vi "GrapFramesRollingBuffer.vi"(0 "object in":refnum<class "Hamamatsu.lvclass">, 5 "error in (no error)":errorcluster) -> (14 "object out":refnum<class "Hamamatsu.lvclass">, 19 "error out":errorcluster)   [LabVIEW 2019, in "Hamamatsu.lvclass"]
uses:
  Hamamatsu.lvclass
  Hamamatsu.lvclass/Hamamatsu.ctl
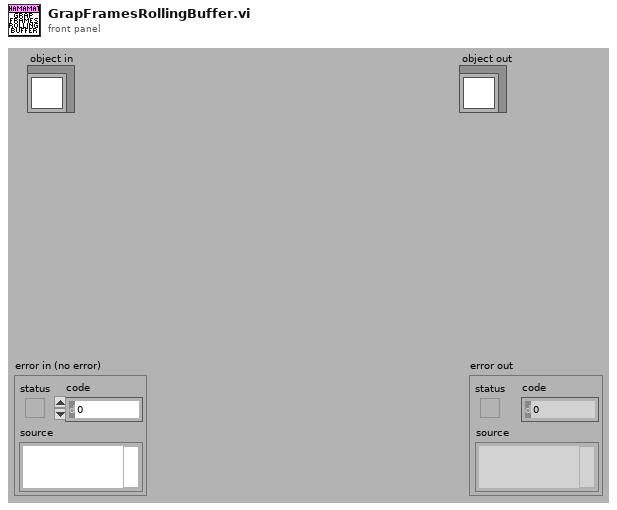
[diagram p1: front panel]
types:
  T1 = typedef "IMAQ Image.ctl" = refnum<image>
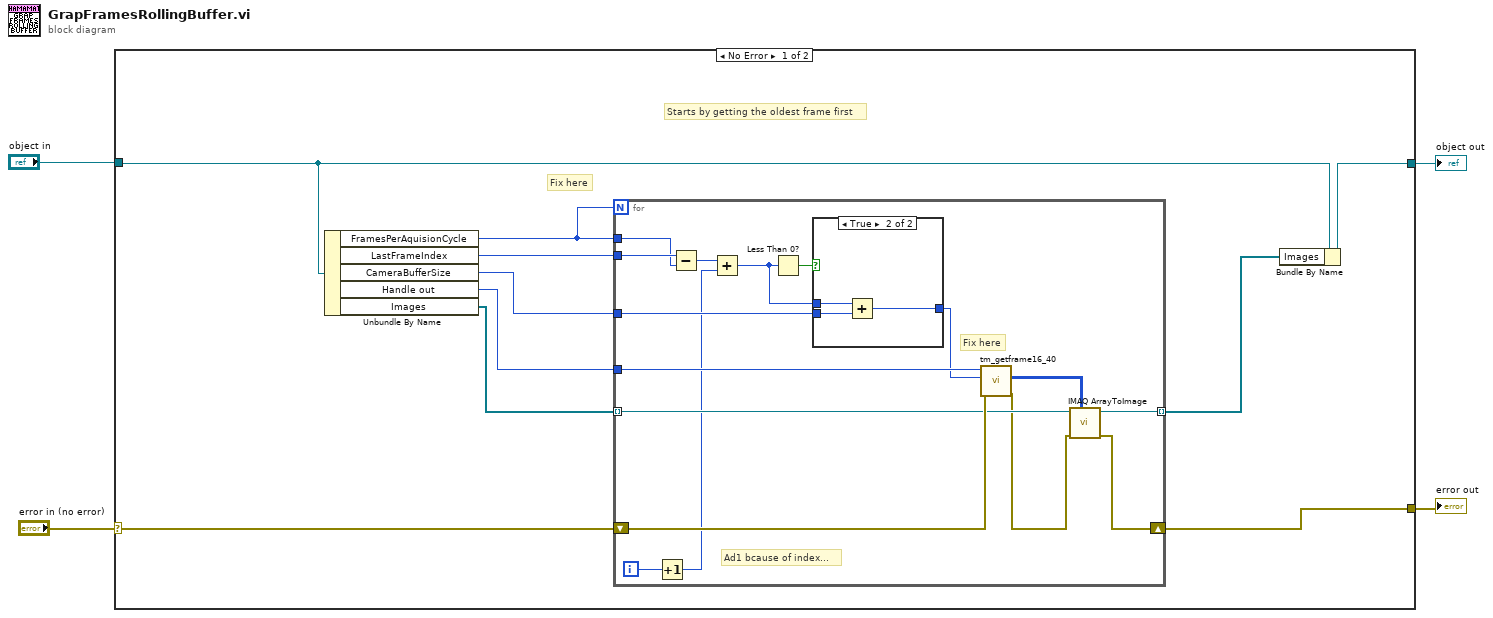
[diagram p0: block diagram]
diagram:
  n1 = case shown="No Error" "error in (no error)" {
    selector: "error in (no error)" -> [w13 w36]
    tunnel: [w12 w36] -> w3
    tunnel: [w14 w35] -> w1
    tunnel: "object in" -> [w11 w35]
    frame No Error {
      # "Starts by getting the oldest frame first"
      # "Fix here"
      n2 = Unbundle By Name(w11) -> ("FramesPerAquisionCycle"=w5:i32, "LastFrameIndex"=w9:i32, "CameraBufferSize"=w8:i32, "Handle out"=w7:u32, "Images"=w6:T1[])
      n3 = for {
        N: w5 -> [_]
        shift-right: [w23] -> w12
        shift-left: w13 -> [w30]
        tunnel: w9 -> [w19]
        tunnel: w5 -> [w17]
        tunnel: w8 -> [w29]
        tunnel: w7 -> [w27]
        tunnel: w6 -> [w25] mode=indexing
        tunnel: [w22] -> w10 mode=indexing
        i -> [w16]
        # "Ad1 bcause of index..."
        # "Fix here"
        n4 = Increment(x=w16) -> (x+1=w15:i32)
        n5 = Subtract(x=w19, y=w17) -> (x-y=w21:i32)
        n6 = Add(x=w21, y=w15) -> (x+y=w20:i32)
        n7 = Less Than 0?(x=w20) -> (x < 0?=w28:bool)
        n8 = case shown="True" w28 {
          tunnel: w29 -> [_ w34]
          tunnel: w20 -> [w31 w33]
          tunnel: [w31 w32] -> w18
          frame False {
          }
          frame True {
            n9 = Add(x=w33, y=w34) -> (x+y=w32:i32)
          }
        }
        n10 = call <userlib>:"tm_getframe16_40.vi"("error in (no error)"=w30, "Frame Index"=w18, "Handle in"=w27) -> ("error out"=w24:errorcluster, "Data"=w26:u16[][])  [unwired: 5 in, 2 out]
        n11 = call "IMAQ ArrayToImage"("Image Pixels (U16)"=w26, "error in (no error)"=w24, "Image"=w25) -> ("error out"=w23:errorcluster, "Image Out"=w22:T1)  [unwired: 7 in]
      }
      n12 = Bundle By Name(cluster=w11, "Images"=w10) -> (w14:refnum<class "Hamamatsu.lvclass">)
    }
    frame Error {
    }
  }
  "error out" <- w3
  "object out" <- w1
